vi "ReadConfig.vi"(8 "error in (no error)":errorcluster, 11 "RoomAlert in":refnum<class "RoomAlert.lvclass">) -> (0 "error out":errorcluster, 2 "Config":variant, 3 "RoomAlert out":refnum<class "RoomAlert.lvclass">)   [LabVIEW 2018, in "SensorPlugins.lvlib" / "RoomAlert.lvclass"]
doc: "Reads all the elements in the configuration cluster."
uses:
  RoomAlert.lvclass
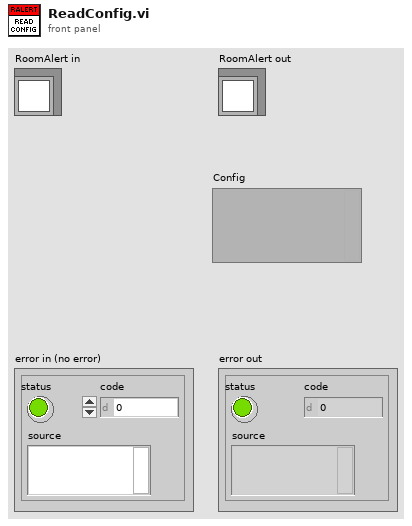
[diagram p1: front panel]
types:
  T1 = typedef "SensorPlugins.lvlib/RoomAlert.lvclass/RoomAlertControls.ctl" = cluster{"Connected?":bool, "IP Address of SNMP Device":string, "Port (161)":u16, "Community Name":string, "Measurements To Read Array":u16[], "Update LightTower?":bool, "LightTower":cluster{"Red":bool, "Amber":bool, "Green":bool, "Audio":bool}, "RoomAlert Model ID":string, "Sensor OID Numbers":string[][], "Sensor Light Tower OID Numbers":string[][]}[]
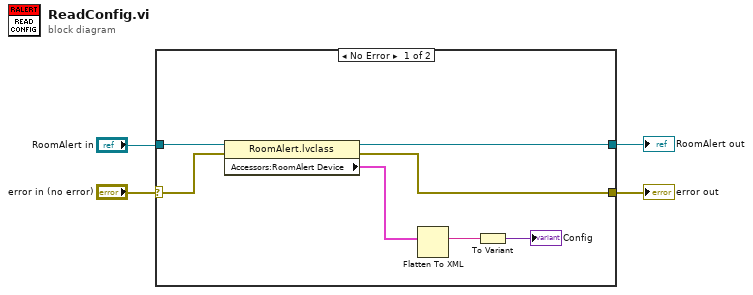
[diagram p0: block diagram]
diagram:
  n1 = case shown="No Error" "error in (no error)" {
    selector: "error in (no error)" -> [w9 w13]
    tunnel: "RoomAlert in" -> [w11 w12]
    tunnel: [w8 w13] -> w1
    tunnel: [w10 w12] -> w2
    frame No Error {
      n2 = property class="RoomAlert.lvclass"(reference=w11, error in=w9) -> (reference out=w10:refnum<class "RoomAlert.lvclass">, error out=w8:errorcluster, "Accessors:RoomAlert Device"=w5:T1)
      n3 = Flatten To XML(anything=w5) -> (xml string=w6:string)
      n4 = To Variant(anything=w6) -> (Variant=→"Config":variant)
    }
    frame Error {
    }
  }
  "error out" <- w1
  "RoomAlert out" <- w2
